vi "Write Transfer Buffer.vi"(8 "error in":errorcluster, 9 "data":u8[](array[numeric]), 10 "Transfer":refnum<class "Transfer.lvclass">, 11 "RDMA Transceiver in":refnum<class "RDMA Transceiver.lvclass">) -> (0 "error out":errorcluster, 3 "RDMA Transceiver out":refnum<class "RDMA Transceiver.lvclass">)   [LabVIEW 2020, in "RDMA.lvlib" / "RDMA Transceiver.lvclass"]
uses:
  RDMA Transceiver.lvclass
  DSF Core.lvlibp/Classes/Transfer/Transfer.lvclass
  Throw Size Mismatch Error.vi
  RDMA Transceiver.lvclass/RDMA Transceiver.ctl
  DSF Core.lvlibp/Classes/Buffer/Buffer.lvclass
  DSF Core.lvlibp/Classes/Buffer/Write Buffer 1D U8.vi
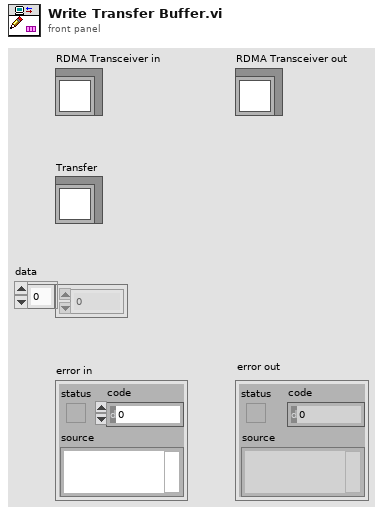
[diagram p1: front panel]
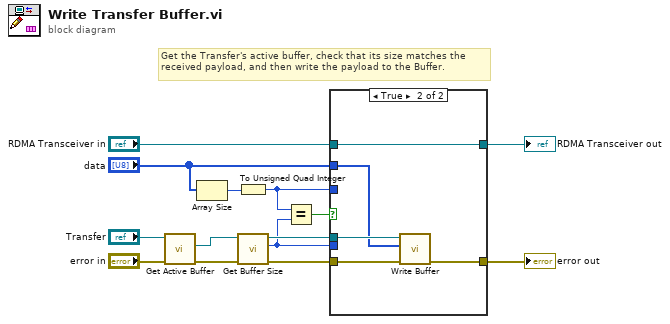
[diagram p0: block diagram]
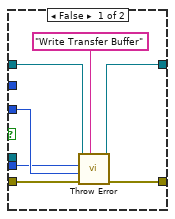
[diagram p2: hidden frame]
diagram:
  # "Get the Transfer's active buffer, check that its size matches the received payload, and then write the payload to the Buffer."
  n1 = call "Get Active Buffer.vi"("error in (no error)"="error in", "Transfer in"="Transfer") -> ("error out"=w5:errorcluster, "Buffer"=w4:refnum<class "Buffer.lvclass">)  [unwired: 7 in, 1 out]
  n2 = Array Size(array="data") -> (size(s)=w13:i32)
  n3 = To Unsigned Quad Integer(1:w13) -> (0:w10:u64)
  n4 = call "Get Buffer Size.vi"("Buffer in"=w4) -> ("buffer size"=w2:u64, "Buffer out"=w12:refnum<class "Buffer.lvclass">)  [unwired: 9 in]
  n5 = Equal?(x=w10, y=w2) -> (x = y?=w11:bool)
  n6 = case shown="True" w11 {
    tunnel: w12 -> [_ w25]
    tunnel: w5 -> [w20 w24]
    tunnel: [w19 w23] -> w3
    tunnel: "RDMA Transceiver in" -> [w18 w22]
    tunnel: [w17 w22] -> w9
    tunnel: w2 -> [w15 _]
    tunnel: w10 -> [w16 _]
    tunnel: "data" -> [_ w21]
    frame False {
      n7 = call-poly "Throw Error.vi"("source vi name"="Write Transfer Buffer", "error in"=w20, "actual size"=w16, "expected size"=w15, "RDMA in"=w18) -> ("error out"=w19:errorcluster, "RDMA out"=w17:refnum<class "RDMA Transceiver.lvclass">)  [unwired: 5 in]
    }
    frame True {
      n8 = call-poly "Write Buffer.vi"("error in (no error)"=w24, "src array in"=w21, "Buffer in"=w25) -> ("error out"=w23:errorcluster)  [unwired: 5 in, 3 out]
    }
  }
  "error out" <- w3
  "RDMA Transceiver out" <- w9
